vi "MEMS_Resistance.vi"() -> ()   [LabVIEW 2017]
panel:
  in  "Tab Control":enum32{"CONTROL", "Reticle Designs", "Data"}(tab)
  in  "READ ACTUATION VOLTAGE FILE?":bool
  in  "stop":bool
  in  "Actuation Voltage File Path":path
  in  "4-Wire Measurement Delay (s)":dbl=0.001
  in  "Actuator Change Delay (s)":dbl=0.001
  in  "Build Array":bool
  in  "Seq4_Enable":bool
  in  "Seq3_Enable":bool
  in  "Seq2_Enable":bool=TRUE
  in  "Seq1_Enable":bool=TRUE
  in  "Actuation Seq 4":string
  in  "Actuation Seq 3":string
  in  "Actuation Seq 2":string="39:0:1"
  in  "Actuation Seq 1":string="0:40:1"
  in  "Compliance Limit (A)":dbl
  in  "Forced Current (A)":dbl
  in  "LCR Measure":bool
  out "LCR Measured Resistance (Ohms)":string="0"
  out "Measured Capacitance (F)":string="0"
  in  "E4981A LCR":refnum<visa-resource-name>="GPIB0::17::INSTR"
  in  "SMU Measure?\nTRUE = SMU\nFALSE = LCR":bool=TRUE
  out "Measured Resistance (Ohms)":string="0"
  in  "Current Limit (A)":dbl=0.1
  in  "Actuation Voltage (V)":dbl
  in  "Actuation Voltage Array (V)":i32[](array[numeric])
  in  "Keithley 2450 SMU":refnum<visa-resource-name>="GPIB0::9::INSTR"
  in  "Keithley 2400 Actuator PS":refnum<visa-resource-name>="GPIB0::3::INSTR"
  out "Measured Current (A)":string="0.106041"
  in  "Error In":errorcluster
  out "Error Out":errorcluster
  in  "Lot#":string="2966C"
  in  "Wafer#":string="04"
  in  "Package":string="BC"
  in  "Base Path":path=path "C:/Wafer Test Data/Minerva1/2966C/AFS/Verify"
  in  "Comment":string="Init"
  in  "Measure Resistance":bool
  in  "Set Actuation Voltage":bool
  in  "TP":string="WRL1 Cascade Prober MEMS Resistance vs Actuation Voltage Sweep Ver1.0"
  in  "Die Selection":bool[][](array[boolean])=[[FALSE, FALSE, FALSE, FALSE, FALSE, FALSE, FALSE, FALSE, FALSE], [FALSE, FALSE, FALSE, FALSE, FALSE, FALSE, FALSE, FALSE, FALSE], [FALSE, FALSE, FALSE, FALSE, FALSE, FALSE, FALSE, FALSE, FALSE], [FALSE, FALSE, FALSE, FALSE, FALSE, FALSE, FALSE, FALSE, FALSE], [FALSE, FALSE, FALSE, FALSE, FALSE, FALSE, FALSE, FALSE, FALSE], [FALSE, FALSE, FALSE, FALSE, FALSE, FALSE, FALSE, FALSE, FALSE], [FALSE, FALSE, TRUE, FALSE, FALSE, FALSE, FALSE, FALSE, FALSE], [FALSE, FALSE, TRUE, FALSE, FALSE, FALSE, FALSE, FALSE, FALSE], [FALSE, FALSE, TRUE, FALSE, FALSE, FALSE, FALSE, FALSE, FALSE]]
  in  "DIEs":u8[](array[numeric])=[1]
  in  "Number of \nReticles":i32=17
  in  "TypeOfTest":u16(ring) items=["Normal", "DML", "TTBD"]
  in  "Start Testing":bool
  in  "Stop Test":bool
  in  "Set Chuck Position":string="0 1 13 "
  out "Status":string="Now Testing... -1 2 0"
  out "Current Position":string="End of wafer -- StepNext"
  out "Table":string[][](table)=[["2966C", "02", "Var", "Init Full", "5/13/2020", "22:00:38", "1 3", "46", "1", "3", "0.094725", "", "CMin", "0", "35.00", "45.051115", "", "0.629833", "44.936020", "", "0.629764", "629.764000E-3", "0.250", "251.905600E+0", "-69.000000E-6", "2000"], ["2966C", "02", "Var", "Init Full", "5/13/2020", "22:00:38", "1 3", "46", "1", "3", "0.094725", "", "TB1", "1", "35.00", "45.099016", "", "0.826441", "45.425674", "", "0.629630", "196.811000E-3", "0.250", "78.724400E+0", "-134.000000E-6", "2000"], ["2966C", "02", "Var", "Init Full", "5/13/2020", "22:00:38", "1 3", "46", "1", "3", "0.094725", "", "TB2", "2", "35.00", "45.202801", "", "0.826375", "45.176827", "", "0.629278", "197.097000E-3", "0.250", "78.838800E+0", "-352.000000E-6", "2000"], ["2966C", "02", "Var", "Init Full", "5/13/2020", "22:00:39", "1 3", "46", "1", "3", "0.094725", "", "TB3", "3", "35.00", "45.766275", "", "0.822180", "45.002521", "", "0.629324", "192.856000E-3", "0.250", "77.142400E+0", "46.000000E-6", "2000"], ["2966C", "02", "Var", "Init Full", "5/13/2020", "22:00:39", "1 3", "46", "1", "3", "0.094725", "", "TB4", "4", "35.00", "45.352464", "", "0.820607", "45.735672", "", "0.630275", "190.332000E-3", "0.250", "76.132800E+0", "951.000000E-6", "2000"], ["2966C", "02", "Var", "Init Full", "5/13/2020", "22:00:39", "1 3", "46", "1", "3", "0.094725", "", "TB5", "5", "35.00", "45.432299", "", "0.850752", "45.159530", "", "0.630097", "220.655000E-3", "0.250", "88.262000E+0", "-178.000000E-6", "2000"], ["2966C", "02", "Var", "Init Full", "5/13/2020", "22:00:40", "1 3", "46", "1", "3", "0.094725", "", "FB3", "6", "35.00", "45.061732", "", "0.738751", "45.192129", "", "0.630700", "108.051000E-3", "0.125", "86.440800E+0", "603.000000E-6", "2000"], ["2966C", "02", "Var", "Init Full", "5/13/2020", "22:00:40", "1 3", "46", "1", "3", "0.094725", "", "FB1", "7", "35.00", "45.339158", "", "0.678171", "45.175497", "", "0.629570", "48.601000E-3", "0.03125", "155.523200E+0", "-1.130000E-3", "2000"]]
  # "Actuation Voltage Definition"
  # "3"
  # "1"
  # "5"
  # "7"
  # "9"
  # "6"
  # "5"
  # "4"
  # "3"
  # "2"
  # "1"
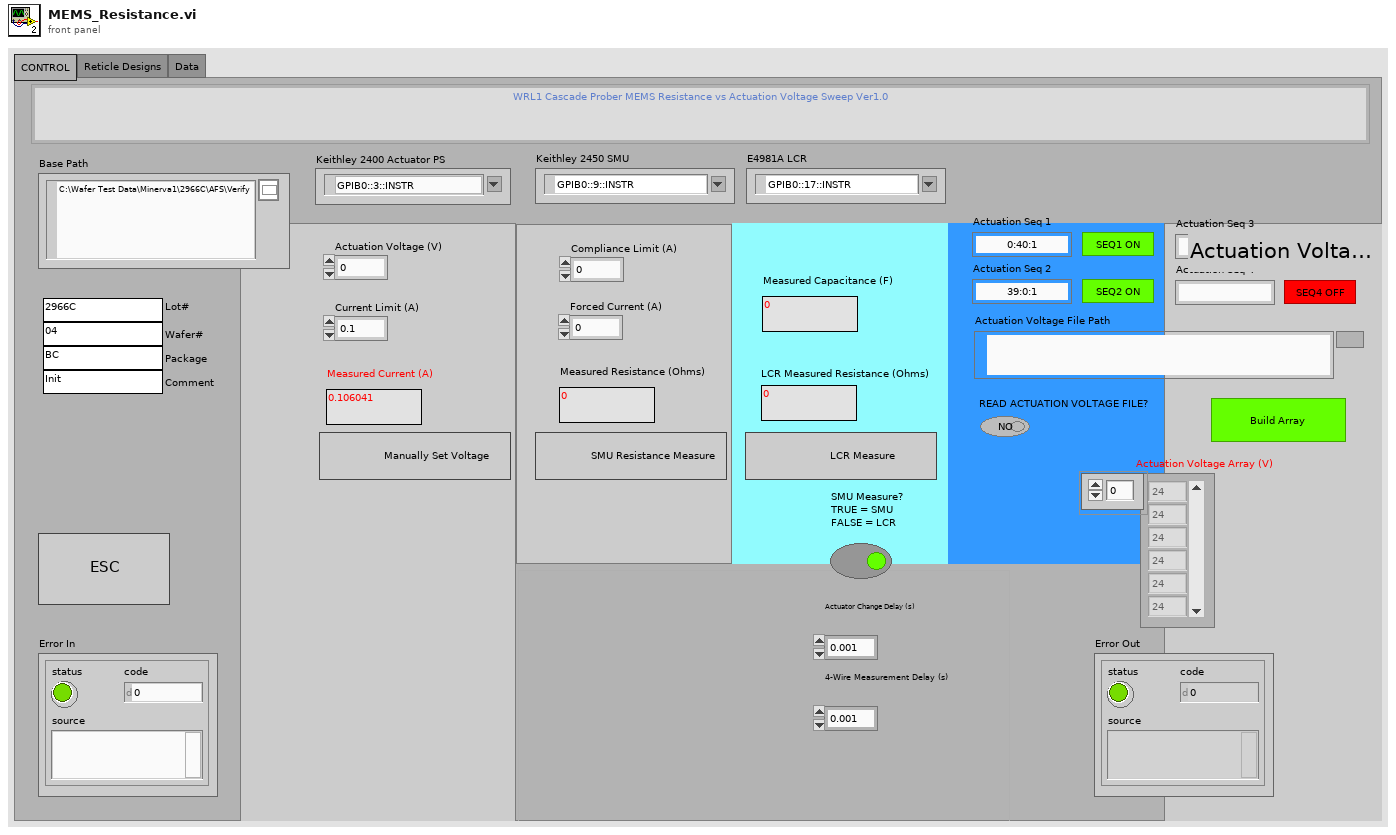
[diagram p1: front panel]
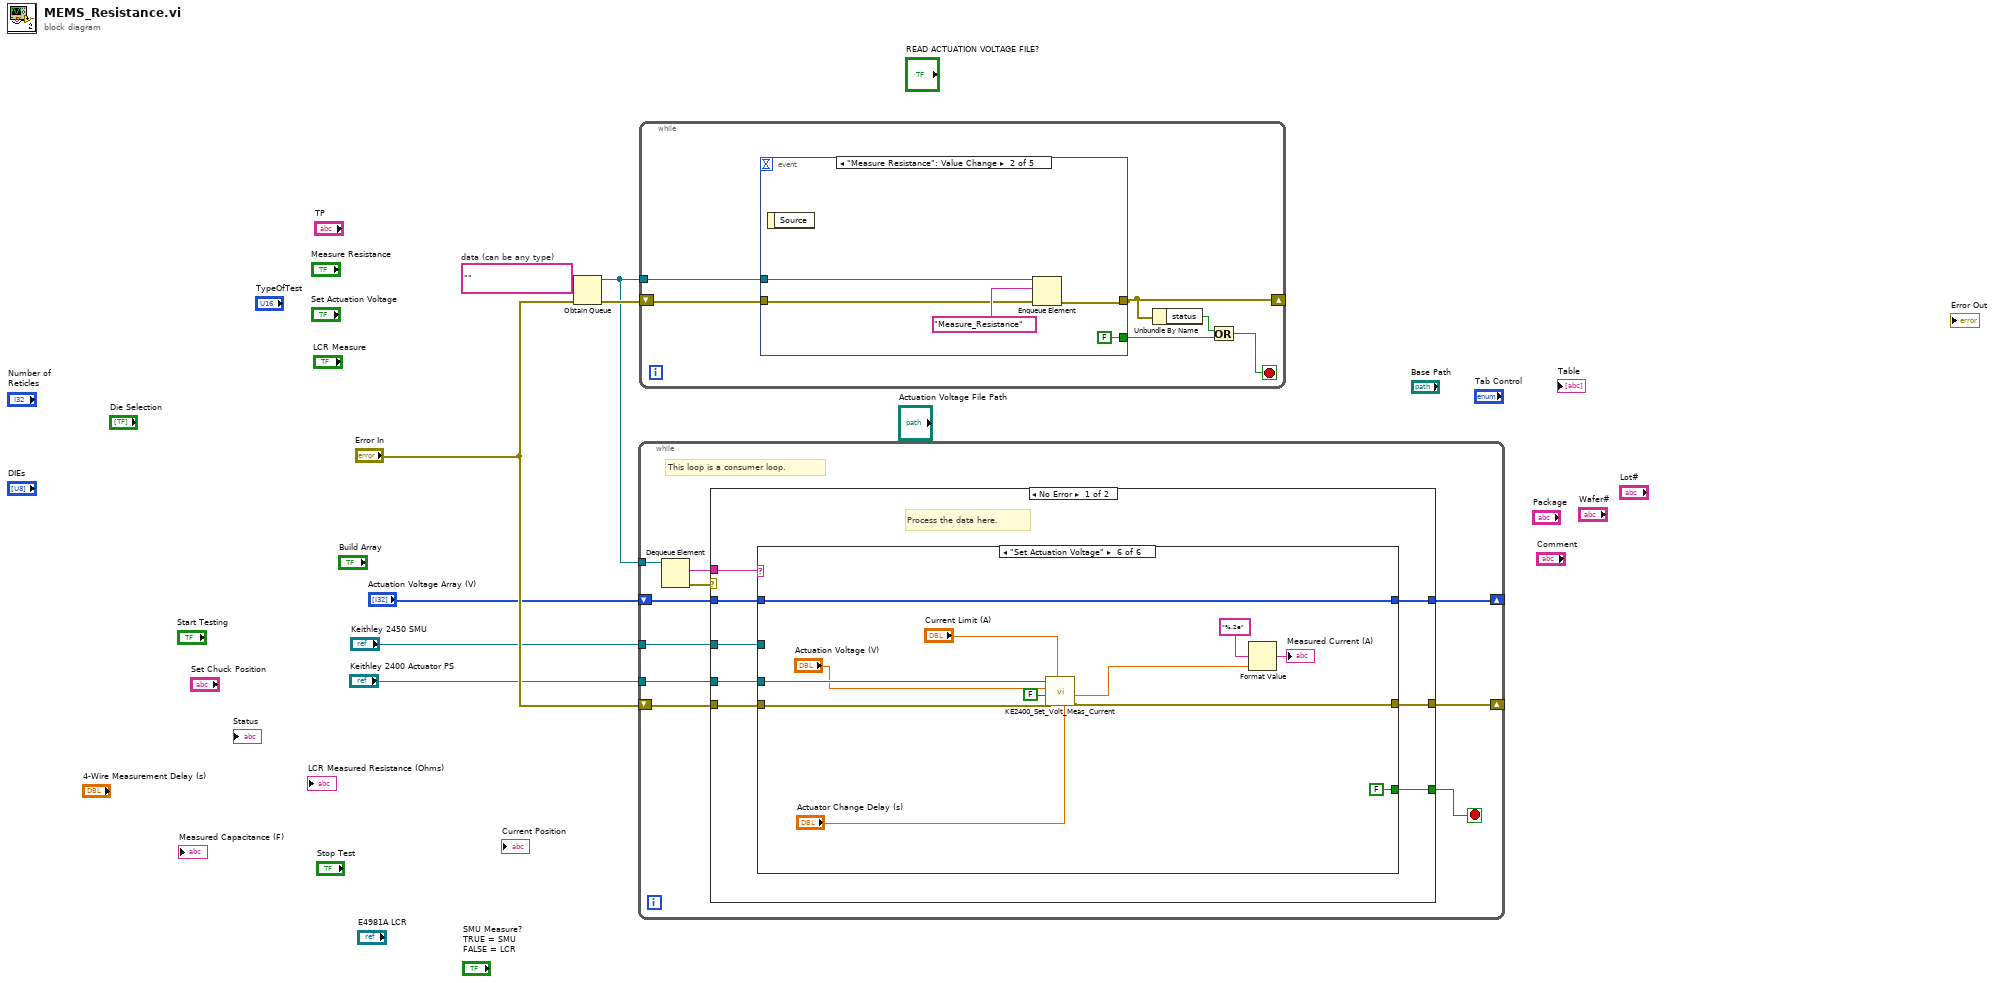
[diagram p0: block diagram]
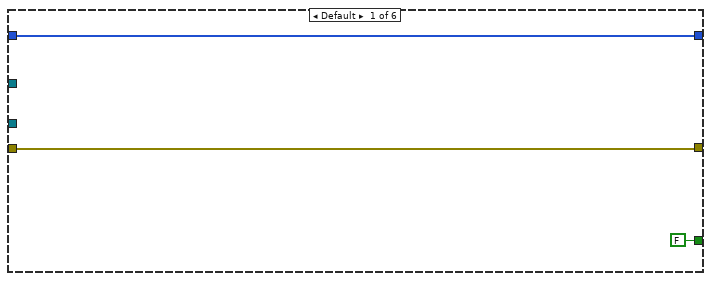
[diagram p2: hidden frame]
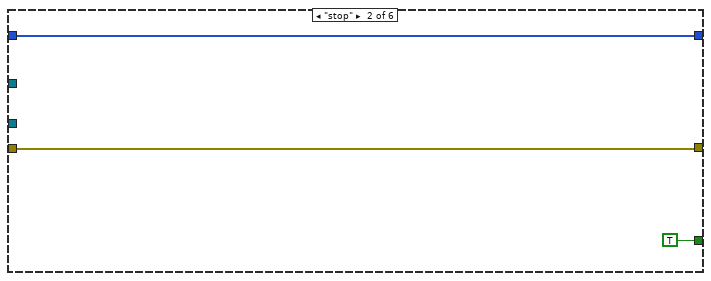
[diagram p3: hidden frame]
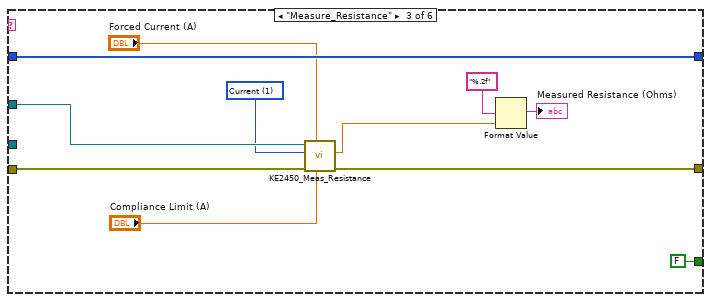
[diagram p4: hidden frame]
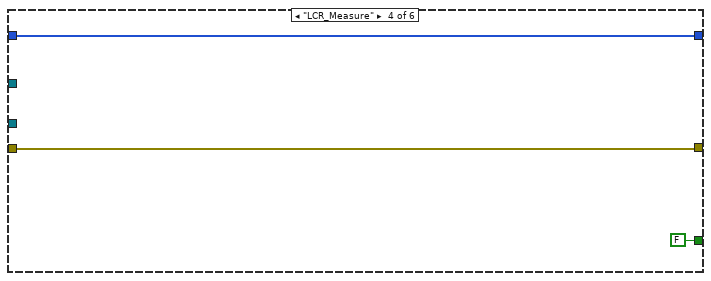
[diagram p5: hidden frame]
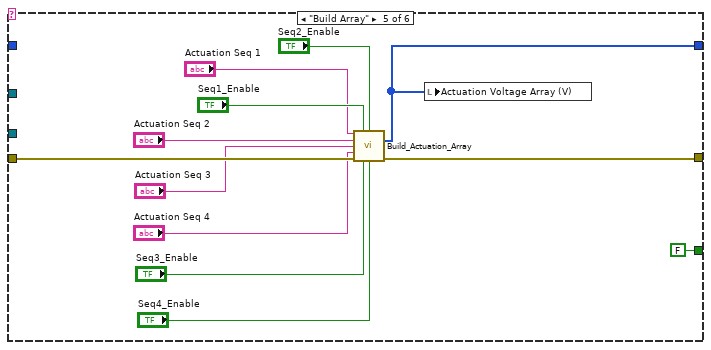
[diagram p6: hidden frame]
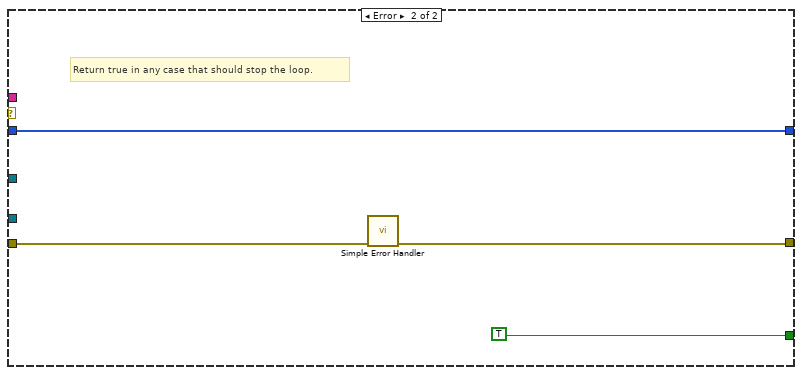
[diagram p7: hidden frame]
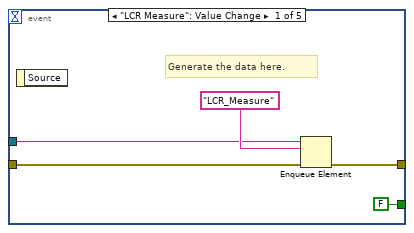
[diagram p8: hidden frame]
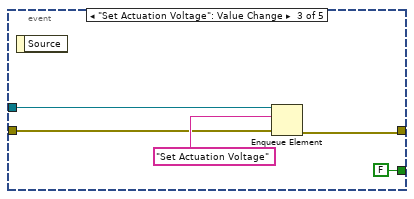
[diagram p9: hidden frame]
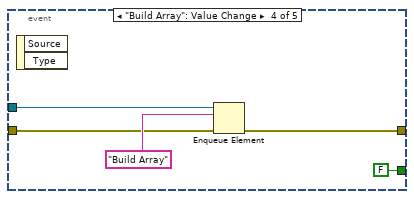
[diagram p10: hidden frame]
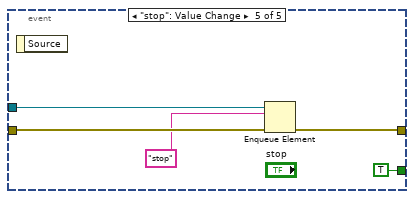
[diagram p11: hidden frame]
diagram:
  w7 = ""  # data (can be any type)
  n1 = Obtain Queue(element data type=w7, error in (no error)="Error In") -> (queue out=w5:refnum<queue>, error out=w6:errorcluster)  [unwired: 3 in, 1 out]
  n2 = while {
    tunnel: w5 -> [w17]
    shift-right: [w11] -> _
    shift-left: "Error In" -> [w13]
    tunnel: "Keithley 2400 Actuator PS" -> [w12]
    shift-right: [w9] -> _
    shift-left: "Actuation Voltage Array (V)" -> [w10]
    tunnel: "Keithley 2450 SMU" -> [w8]
    stop <- w14 stop-if-true
    # "This loop is a consumer loop."
    n3 = Dequeue Element(queue=w17) -> (element=w15:string, error out=w16:errorcluster)  [unwired: 2 in, 2 out]
    n4 = case shown="No Error" w16 {
      tunnel: w15 -> [w25 _]
      tunnel: [w18 TRUE] -> w14
      tunnel: w13 -> [w24 w71]
      tunnel: w12 -> [w23 _]
      tunnel: [w22 w70] -> w11
      tunnel: w10 -> [w20 w72]
      tunnel: [w21 w72] -> w9
      tunnel: w8 -> [w19 _]
      frame No Error {
        # "Process the data here."
        n5 = case shown="\"Set Actuation Voltage\"" w25 {
          tunnel: w24 -> [w28 w30 w39 w45 w57 w65]
          tunnel: w23 -> [_ _ _ _ _ w63]
          tunnel: [w28 w30 w38 w45 w56 w59] -> w22
          tunnel: w20 -> [w27 w31 w42 w44 _ w67]
          tunnel: [w27 w31 w42 w44 w47 w67] -> w21
          tunnel: w19 -> [_ _ w37 _ _ _]
          tunnel: [FALSE TRUE FALSE FALSE FALSE FALSE] -> w18
          frame Default {
          }
          frame "stop" {
          }
          frame "Measure_Resistance" {
            w36 = u16 1 items=["Voltage", "Current"] ("Source Mode  (0: Voltage)")
            n6 = call "KE2450_Meas_Resistance.vi"("Compliance Level (0.1)"="Compliance Limit (A)", "Output Level (0)"="Forced Current (A)", "error in (no error)"=w39, "Source Mode  (0: Voltage)"=w36, "VISA resource name"=w37) -> ("error out"=w38:errorcluster, "Resistance (ohm)"=w33:dbl)  [unwired: 3 in, 2 out]
            n7 = Format Value(format string="%.2f", value (0)=w33) -> (output string=→"Measured Resistance (Ohms)":string)  [unwired: 1 in]
          }
          frame "LCR_Measure" {
          }
          frame "Build Array" {
            n8 = call "Build_Actuation_Array.vi"("Actuation Seq 1"="Actuation Seq 1", "Seq1_Enable"="Seq1_Enable", "Seq2_Enable"="Seq2_Enable", "Actuation Seq 2"="Actuation Seq 2", "Actuation Seq 3"="Actuation Seq 3", "Actuation Seq 4"="Actuation Seq 4", "error in (no error)"=w57, "Seq3_Enable"="Seq3_Enable", "Seq4_Enable"="Seq4_Enable") -> ("Array Out"=w47:i32[], "error out"=w56:errorcluster)  [unwired: 5 in]
            n9 = local write "Actuation Voltage Array (V)"(w47) -> ()
          }
          frame "Set Actuation Voltage" {
            n10 = call "KE2400_Set_Volt_Meas_Current.vi"("Manual Settling Delay (0 sec)"="Actuator Change Delay (s)", "Compliance  Level (0.1)"="Current Limit (A)", "error in (no error)"=w65, "Enable Remote Sensing (T: Enable)"=FALSE, "Output Level (0)"="Actuation Voltage (V)", "VISA resource name"=w63) -> ("error out"=w59:errorcluster, "Current"=w64:sgl)  [unwired: 3 in, 1 out]
            n11 = Format Value(format string="%.2e", value (0)=w64) -> (output string=→"Measured Current (A)":string)  [unwired: 1 in]
          }
        }
      }
      frame Error {
        # "Return true in any case that should stop the loop."
        n12 = call <vilib>:"Simple Error Handler.vi"("error in (no error)"=w71) -> ("error out"=w70:errorcluster)  [unwired: 4 in, 4 out]
      }
    }
  }
  n13 = while {
    shift-right: [w77] -> _
    shift-left: w6 -> [w79]
    tunnel: w5 -> [w76]
    stop <- w74 stop-if-true
    n14 = event shown="[1] \"Measure Resistance\": Value Change" {
      selector: _ -> [_ _ _ _ _]
      dyn-events: _ -> [_ _ _ _ _]
      timeout: _ -> [_ _ _ _ _]
      tunnel: w79 -> [w83 w88 w93 w98 w103]
      tunnel: [w82 w87 w92 w96 w104] -> w77
      tunnel: w76 -> [w81 w86 w91 w97 w102]
      tunnel: [FALSE ("stop") FALSE ("stop") FALSE ("stop") FALSE ("stop") TRUE ("stop")] -> w75
      event "LCR Measure": Value Change {
        # "Generate the data here."
        n15 = event-data() -> ()  [unwired: 1 in, 1 out]
        n16 = Enqueue Element(queue=w81, element="LCR_Measure", error in (no error)=w83) -> (error out=w82:errorcluster)  [unwired: 1 in, 2 out]
      }
      event "Measure Resistance": Value Change {
        n17 = event-data() -> ()  [unwired: 1 in, 1 out]
        n18 = Enqueue Element(queue=w86, element="Measure_Resistance", error in (no error)=w88) -> (error out=w87:errorcluster)  [unwired: 1 in, 2 out]
      }
      event "Set Actuation Voltage": Value Change {
        n19 = event-data() -> ()  [unwired: 1 in, 1 out]
        n20 = Enqueue Element(queue=w91, element="Set Actuation Voltage", error in (no error)=w93) -> (error out=w92:errorcluster)  [unwired: 1 in, 2 out]
      }
      event "Build Array": Value Change {
        n21 = event-data() -> ()  [unwired: 1 in, 2 out]
        n22 = Enqueue Element(queue=w97, element="Build Array", error in (no error)=w98) -> (error out=w96:errorcluster)  [unwired: 1 in, 2 out]
      }
      event "stop": Value Change {
        n23 = event-data() -> ()  [unwired: 1 in, 1 out]
        n24 = Enqueue Element(queue=w102, element="stop", error in (no error)=w103) -> (error out=w104:errorcluster)  [unwired: 1 in, 2 out]
      }
    }
    n25 = Unbundle By Name(w77) -> ("status"=w78:bool)
    n26 = Or(x=w78, y=w75) -> (x .or. y?=w74:bool)
  }
